vi "DIAdem Request Query_test.vi"(8 "error in (no error)":errorcluster, 9 "Username (empty)":string, 11 "Query TDM":path) -> (0 "error out":errorcluster, 3 "Generated Report Path":path)   [LabVIEW 2011]
uses:
  DIAdem Daemon Queue.ctl
  DIAdem Daemon Script Type.ctl
  server lib/Spartan Object Types.ctl
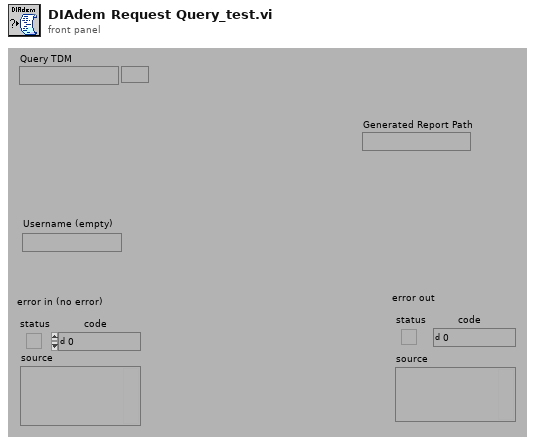
[diagram p1: front panel]
types:
  T1 = typedef "Spartan Object Types.ctl" = enum16{"System", "Test", "Test Config", "Test Storage", "Driver", "Driver Config", "CGI", "CGI Language", "Report Config", "Test Version", "Driver Version", "System Version", "Client Version", "Test Pre-Process", "Unflatten Test Parameters", "Flatten Test Parameters"}
  T2 = typedef "DIAdem Daemon Script Type.ctl" = enum16{"Report", "Query", "Script", "Datasheet", "Append", "Restart", "Stop"}
  T3 = typedef "DIAdem Daemon Queue.ctl" = cluster{"Report Template TDM":path, "Report Processor VBS":path, "Report Path PDF":path, "Report Script Params":string, "Username":string, "Script Type":T2, "Report Query Params":string, "Client Machine":string, "Print on Client?":bool, "Response Queue Name":string, "Script Variables":string[], "Start Request Time":timestamp, "Wait?":bool}
  T4 = typedef "DIAdem Reference.ctl" = cluster{"ToCommand Reference":refnum<k7>, "ToDataSheet Reference":refnum<k7>}
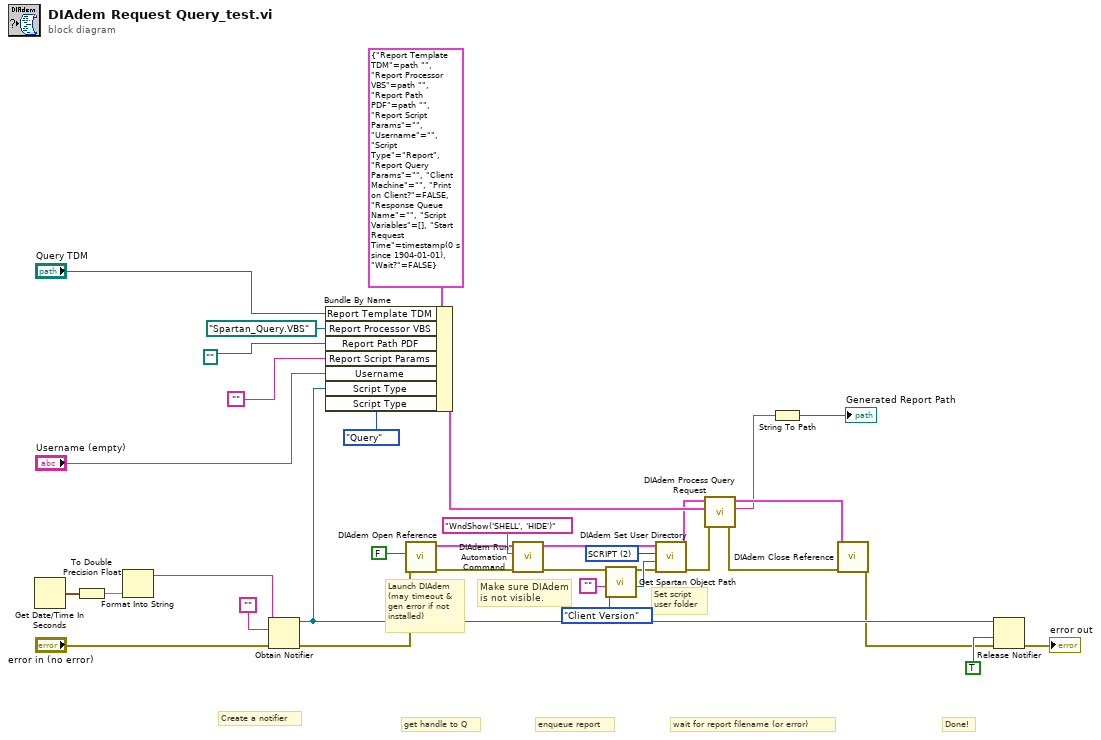
[diagram p0: block diagram]
diagram:
  w16 = u16 2 items=["NAVIGATOR", "REPORT", "SCRIPT"] ("DIAdem panel")
  # "Make sure DIAdem\nis not visible."
  # "Launch DIAdem\n(may timeout &\ngen error if not\ninstalled)"
  # "Set script\nuser folder"
  # "Done!"
  # "wait for report filename (or error)"
  # "enqueue report"
  # "get handle to Q"
  # "Create a notifier"
  n1 = Get Date/Time In Seconds() -> (seconds since 1Jan1904=w33:timestamp)
  n2 = To Double Precision Float(number=w33) -> (double precision float=w32:dbl)
  n3 = Format Into String(w32) -> (resulting string=w31:string)  [unwired: 3 in, 1 out]
  n4 = Obtain Notifier(name (unnamed)=w31, notification data type="", error in (no error)="error in (no error)") -> (notifier out=w20:refnum<notifier>, error out=w7:errorcluster)  [unwired: 1 in, 1 out]
  n5 = Bundle By Name(cluster=T3 {"Report Template TDM"=path "", "Report Processor VBS"=path "", "Report Path PDF"=path "", "Report Script Params"="", "Username"="", "Script Type"=enum."Report", "Report Query Params"="", "Client Machine"="", "Print on Client?"=FALSE, "Response Queue Name"="", "Script Variables"=[], "Start Request Time"=timestamp(0 s since 1904-01-01), "Wait?"=FALSE} ("DD_Report"), "Report Template TDM"="Query TDM", "Report Processor VBS"=path "Spartan_Query.VBS", "Report Path PDF"=path "", "Report Script Params"="", "Username"="Username (empty)", "Script Type"=w20, "Script Type"=DIAdem_Daemon_Script_Type."Query") -> (w19:T3)
  n6 = call <vilib>:"DIAdem Open Reference.vi"("error in (no error)"=w7, "Show Environment (F)"=FALSE) -> ("error out"=w11:errorcluster, "DIAdem Reference"=w12:T4)  [unwired: 8 in]
  n7 = call <vilib>:"DIAdem Run Automation Command.vi"("error in (no error)"=w11, "command"="WndShow('SHELL', 'HIDE')", "DIAdem Reference"=w12) -> ("error out"=w9:errorcluster, "DIAdem Reference"=w10:T4)  [unwired: 7 in]
  n8 = call "Get Spartan Object Path.vi"("Object Type (Test Config)"=Spartan_Object_Types."Client Version", "Object Name (\"\")"="") -> ("Object Path"=w15:path)  [unwired: 8 in, 1 out]
  n9 = call <vilib>:"DIAdem Set User Directory.vi"("error in (no error)"=w9, "user directory"=w15, "DIAdem panel"=w16, "DIAdem Reference"=w10) -> ("error out"=w6:errorcluster, "DIAdem Reference"=w8:T4)  [unwired: 6 in]
  n10 = call "DIAdem Process Query Request.vi"("error in (no error)"=w6, "DIAdem Queue"=w19, "DIAdem Reference"=w8) -> ("error out"=w5:errorcluster, "Results"=w2:string, "dup DIAdem Reference"=w4:T4)  [unwired: 3 in]
  n11 = String To Path(string=w2) -> (path=→"Generated Report Path":path)
  n12 = call <vilib>:"DIAdem Close Reference.vi"("error in (no error)"=w5, "DIAdem Reference"=w4) -> ("error out"=w3:errorcluster)  [unwired: 9 in]
  n13 = Release Notifier(notifier=w20, force destroy? (F)=TRUE, error in (no error)=w3) -> (error out=→"error out":errorcluster)  [unwired: 2 out]
